vi "LoadBufferForMultiListBoxAndFormat.vi"(6 "MCListbox Refnum":refnum<vi>, 7 "configuration in":T1, 8 "error in (no error)":errorcluster, 9 "channel names in":string[](array[string]), 10 "group names in":string[](array[string]), 11 "tdms file in":refnum<k34>) -> (0 "error out":errorcluster, 3 "tdms file out":refnum<k34>)   [LabVIEW 2017]
uses:
  <vilib>/Utility/tdmsutil.llb/fileViewerConfigData.ctl
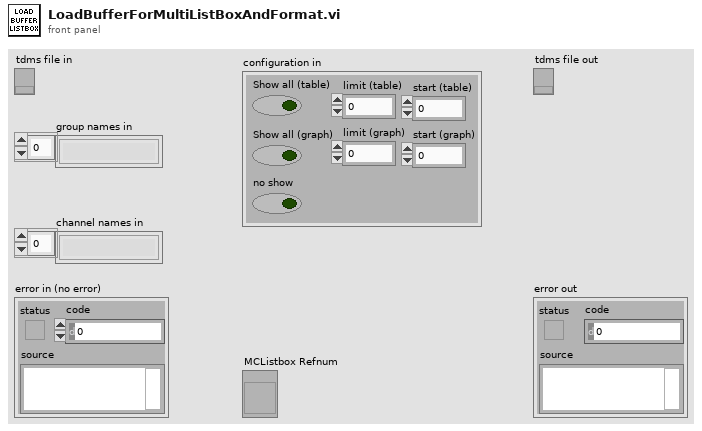
[diagram p1: front panel]
types:
  T1 = typedef "fileViewerConfigData.ctl" = cluster{"Show all (table)":bool, "Show all (graph)":bool, "limit (table)":u64, "limit (graph)":u64, "no show":bool, "start (table)":u64, "start (graph)":u64}
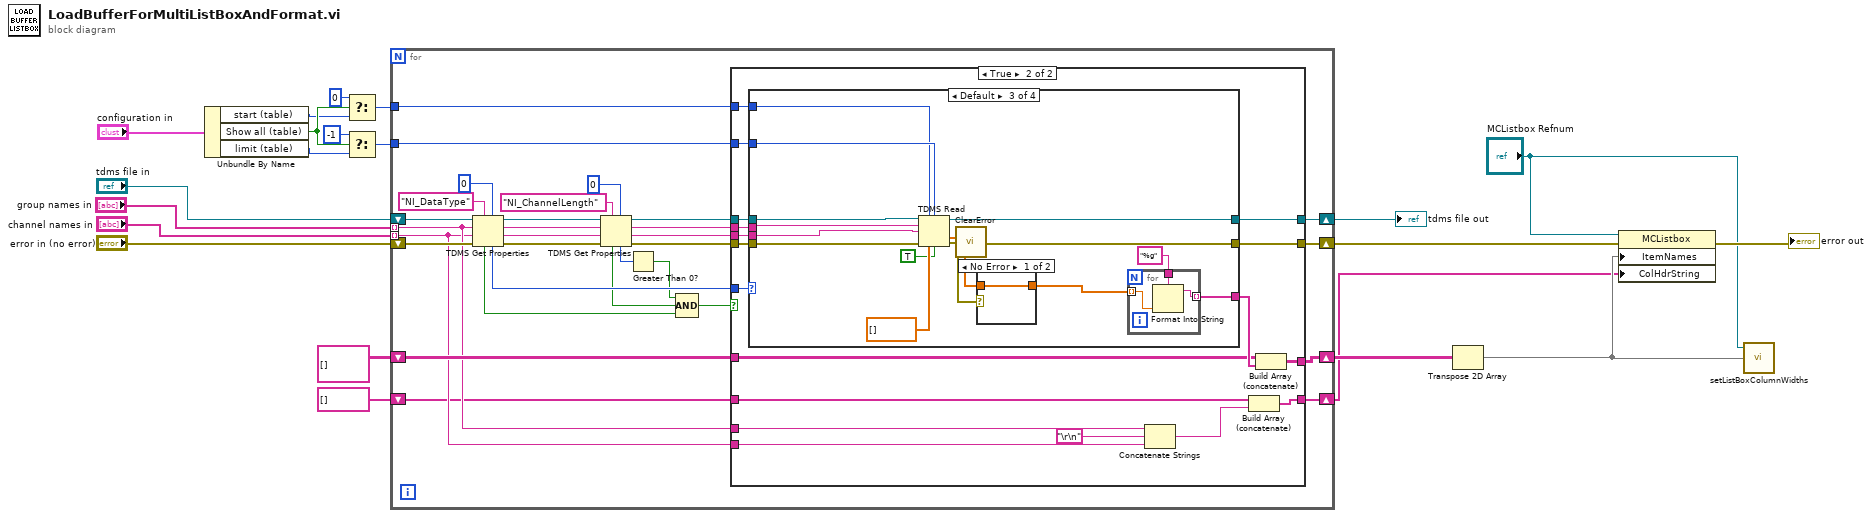
[diagram p0: block diagram]
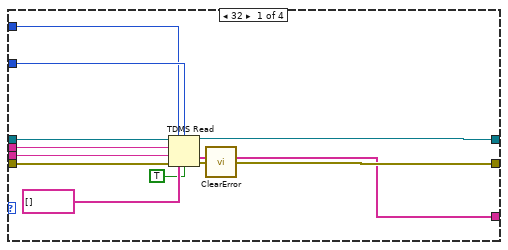
[diagram p3: hidden frame]
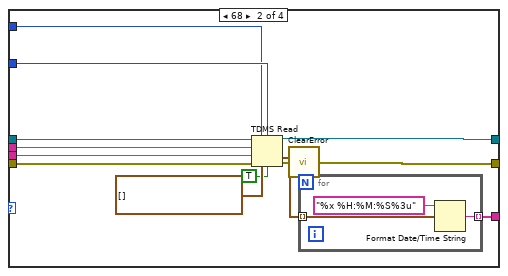
[diagram p4: hidden frame]
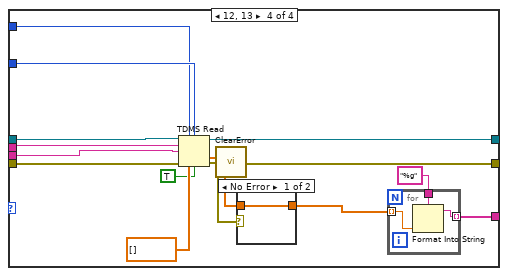
[diagram p6: hidden frame]
diagram:
  n1 = Unbundle By Name("configuration in") -> ("start (table)"=w16:u64, "Show all (table)"=w17:bool, "limit (table)"=w18:u64)
  n2 = Select(t=u64 0, s=w17, f=w16) -> (s? t:f=w19:u64)
  n3 = Select(t=i64 -1 ("count (-1: all)"), s=w17, f=w18) -> (s? t:f=w20:u64)
  n4 = for {
    tunnel: "channel names in" -> [w24] mode=indexing
    shift-right: [w50] -> w3
    shift-left: "error in (no error)" -> [w49]
    shift-right: [w51] -> w10
    shift-left: "tdms file in" -> [w48]
    tunnel: "group names in" -> [w25] mode=indexing
    tunnel: w20 -> [w44]
    tunnel: w19 -> [w43]
    shift-right: [w26] -> w8
    shift-left: string[][] [] -> [w27]
    shift-right: [w22] -> w4
    shift-left: string[] [] -> [w23]
    n5 = TDMS Get Properties(5:u16 0, 7:"NI_DataType" ("property name"), 8:w49, 9:w24, 10:w25, 11:w48) -> (0:w42:errorcluster, 1:w35:string, 2:w36:string, 3:w41:refnum<k34>, 4:w45:u16, 6:w29:bool)
    n6 = TDMS Get Properties(5:u64 0, 7:"NI_ChannelLength" ("property name"), 8:w42, 9:w35, 10:w36, 11:w41) -> (0:w40:errorcluster, 1:w39:string, 2:w38:string, 3:w37:refnum<k34>, 4:w32:u64, 6:w30:bool)
    n7 = Greater Than 0?(x=w32) -> (x > 0?=w31:bool)
    n8 = Compound Arithmetic op=AND(w31, w30, w29) -> (w28:bool)
    n9 = case shown="True" w28 {
      tunnel: [w55 w73] -> w51
      tunnel: [w54 w65] -> w50
      tunnel: w37 -> [w55 w72]
      tunnel: w40 -> [w54 w71]
      tunnel: w38 -> [_ w70]
      tunnel: w39 -> [_ w69]
      tunnel: w45 -> [_ w68]
      tunnel: w44 -> [_ w67]
      tunnel: w43 -> [_ w66]
      tunnel: w27 -> [w53 w62]
      tunnel: [w53 w63] -> w26
      tunnel: w25 -> [_ w60]
      tunnel: w24 -> [_ w56]
      tunnel: w23 -> [w52 w59]
      tunnel: [w52 w57] -> w22
      frame False {
      }
      frame True {
        n10 = case shown="Default" w68 {
          tunnel: [w79 w92 w113 w132] -> w73
          tunnel: [w80 w93 w114 w133] -> w65
          tunnel: [w78 w91 w107 w126] -> w64
          tunnel: w72 -> [w85 w98 w105 w124]
          tunnel: w71 -> [w82 w95 w102 w121]
          tunnel: w70 -> [w84 w97 w104 w123]
          tunnel: w69 -> [w83 w96 w103 w122]
          tunnel: w67 -> [w77 w89 w112 w131]
          tunnel: w66 -> [w76 w88 w111 w130]
          frame 32 {
            n11 = TDMS Read(0:w85, 1:w76, 2:w77, 5:w84, 7:w83, 11:w82, 12:string[] [], 13:TRUE ("return channels in file order? (F)")) -> (4:w79:refnum<k34>, 10:w78:string[], 15:w75:errorcluster)  [unwired: 3 out]
            n12 = call <vilib>:"ClearError.vi"("error in (no error)"=w75) -> ("error out"=w80:errorcluster)
          }
          frame 68 {
            n13 = TDMS Read(0:w98, 1:w88, 2:w89, 5:w97, 7:w96, 11:w95, 12:timestamp[] [], 13:TRUE ("return channels in file order? (F)")) -> (4:w92:refnum<k34>, 10:w90:timestamp[], 15:w87:errorcluster)  [unwired: 3 out]
            n14 = call <vilib>:"ClearError.vi"("error in (no error)"=w87) -> ("error out"=w93:errorcluster)
            n15 = for {
              tunnel: [w101] -> w91 mode=indexing
              tunnel: w90 -> [w100] mode=indexing
              n16 = Format Date/Time String(time format string (%c)="%x %H:%M:%S%3u", seconds (now)=w100) -> (date/time string=w101:string)  [unwired: 1 in]
            }
          }
          frame Default {
            n17 = TDMS Read(0:w105, 1:w111, 2:w112, 5:w104, 7:w103, 11:w102, 12:dbl[] [], 13:TRUE ("return channels in file order? (F)")) -> (4:w113:refnum<k34>, 10:w116:dbl[], 15:w110:errorcluster)  [unwired: 3 out]
            n18 = call <vilib>:"ClearError.vi"("error in (no error)"=w110) -> ("error out"=w114:errorcluster)
            n19 = case shown="No Error" w114 {
              tunnel: w116 -> [w120 _]
              tunnel: [w120 _] -> w108
              frame No Error {
              }
              frame Error {
              }
            }
            n20 = for {
              tunnel: "%g" ("format string") -> [w119]
              tunnel: w108 -> [w118] mode=indexing
              tunnel: [w117] -> w107 mode=indexing
              n21 = Format Into String(format string=w119, w118) -> (resulting string=w117:string)  [unwired: 2 in, 1 out]
            }
          }
          frame 12, 13 {
            n22 = TDMS Read(0:w124, 1:w130, 2:w131, 5:w123, 7:w122, 11:w121, 12:cdb[] [], 13:TRUE ("return channels in file order? (F)")) -> (4:w132:refnum<k34>, 10:w135:cdb[], 15:w129:errorcluster)  [unwired: 3 out]
            n23 = call <vilib>:"ClearError.vi"("error in (no error)"=w129) -> ("error out"=w133:errorcluster)
            n24 = case shown="No Error" w133 {
              tunnel: w135 -> [w139 _]
              tunnel: [w139 _] -> w127
              frame No Error {
              }
              frame Error {
              }
            }
            n25 = for {
              tunnel: "%g" ("format string") -> [w138]
              tunnel: w127 -> [w137] mode=indexing
              tunnel: [w136] -> w126 mode=indexing
              n26 = Format Into String(format string=w138, w137) -> (resulting string=w136:string)  [unwired: 2 in, 1 out]
            }
          }
        }
        n27 = Concatenate Strings(w60, "\r\n", w56) -> (w58:string)
        n28 = Build Array (concatenate)(w59, w58) -> (w57:string[])
        n29 = Build Array (concatenate)(w62, w64) -> (w63:string[][])
      }
    }
  }
  "tdms file out" <- w10
  n30 = Transpose 2D Array(2D array=w8) -> (transposed array=w5:string[][])
  n31 = property on="Property Node" class="MCListbox"(reference="MCListbox Refnum", error in=w3, "ItemNames"=w5, "ColHdrString"=w4) -> (error out=→"error out":errorcluster)  [unwired: 1 out]
  n32 = call <vilib>:"setListBoxColumnWidths.vi"("table data"=w5, "MCListbox Refnum"="MCListbox Refnum") -> ()  [unwired: 1 out]
